vi "ICM Open Query.vi"(8 "error in (no error)":errorcluster, 11 "ICM File In":path) -> (0 "error out":errorcluster, 3 "Query out":refnum<class "Query.lvclass">)   [LabVIEW 2018]
doc: "ICM Open Query.vi\n\nThis VI finds the Query of the current configuration file, opens the object, and reads its configuration data.\n\nInstrument Communication Module Version 1.0\nSeptember, 2017 Original Code Consulting David Thomson\n www.originalcode.com"
uses:
  Query/Query.lvclass
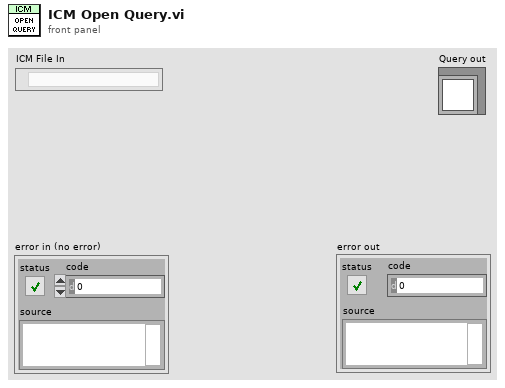
[diagram p1: front panel]
types:
  T1 = enum32{"invalid app kind", "Development System", "Run Time System", "Student Edition", "Embedded LabVIEW", "Evaluation", "Custom"}
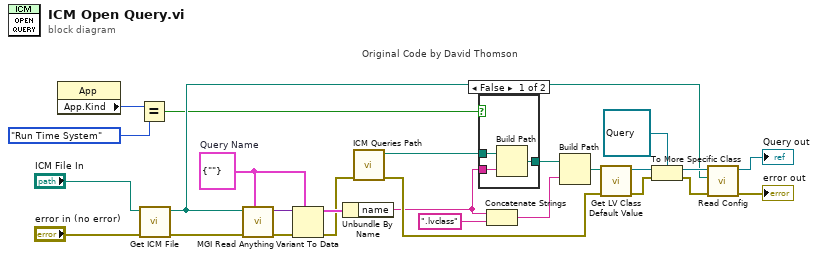
[diagram p0: block diagram]
diagram:
  w24 = cluster{"name":string} {"name"=""}  # Query Name
  n1 = property class="App"() -> ("App.Kind"=w6:T1)  [unwired: 2 in, 2 out]
  n2 = Equal?(x=w6, y=T1."Run Time System" ("Application:Kind")) -> (x = y?=w1:bool)
  n3 = call "Get ICM File.vi"("error in (no error)"="error in (no error)", "ICM File In"="ICM File In") -> ("error out"=w17:errorcluster, "ICM File"=w9:path)  [unwired: 8 in]
  n4 = call <userlib>:"MGI Read Anything.vi"("Type of Anything"=w24, "Error In"=w17, "Path (dialog)"=w9) -> ("Error Out"=w26:errorcluster, "Anything"=w25:variant)  [unwired: 5 in, 2 out]
  n5 = Variant To Data(error in=w26, type=w24, Variant=w25) -> (data=w20:cluster{"name":string}, error out=w8:errorcluster)
  n6 = Unbundle By Name(w20) -> ("name"=w2:string)
  n7 = call "ICM Queries Path.vi"("error in (no error)"=w8) -> ("error out"=w7:errorcluster, "ICM Queries Path"=w4:path)  [unwired: 9 in]
  n8 = case "Original Code by David Thomson" shown="False" w1 {
    tunnel: w4 -> [w29 w30]
    tunnel: [w28 w30] -> w3
    tunnel: w2 -> [w27 _]
    frame False {
      n9 = Build Path(base path=w29, name or relative path=w27) -> (appended path=w28:path)
    }
    frame True {
    }
  }
  n10 = Concatenate Strings(w2, ".lvclass" ("string")) -> (w21:string)
  n11 = Build Path(base path=w3, name or relative path=w21) -> (appended path=w23:path)
  n12 = call <vilib>:"Get LV Class Default Value.vi"("error in (no error)"=w7, "class path"=w23) -> ("error out"=w19:errorcluster, "object"=w18:refnum<class>)  [unwired: 8 in]
  n13 = To More Specific Class(target class=refnum<class "Query.lvclass"> refnum ("Query.lvclass"), reference=w18, error in=w19) -> (specific class reference=w12:refnum<class "Query.lvclass">, error out=w11:errorcluster)
  n14 = call-dynamic "Read Config.vi"("error in (no error)"=w11, "ICM File In"=w9, "Query in"=w12) -> ("error out"=→"error out":errorcluster, "Query out"=→"Query out":refnum<class "Query.lvclass">)  [unwired: 7 in]
